vi "WriteScript.vi"(0 "X1":dbl[](array[numeric]), 1 "Y1":dbl[](array[numeric]), 2 "X2":dbl[](array[numeric]), 3 "Y2":dbl[](array[numeric]), 4 "Pause":i32, 5 "C0":i32, 6 "C1":i32, 7 "error in":errorcluster, 9 "Seq":string) -> (20 "concatenated string":string, 27 "error out":errorcluster)   [LabVIEW 2017]
panel:
  out "B2":dbl
  out "G2":dbl
  out "R2":dbl
  out "Resolved Color 2":u32 format="%.0x"
  out "B1":dbl
  out "G1":dbl
  out "R1":dbl
  out "Resolved Color 1":u32 format="%.0x"
  # "M. Zemp & I. Scholl GM BA 2"
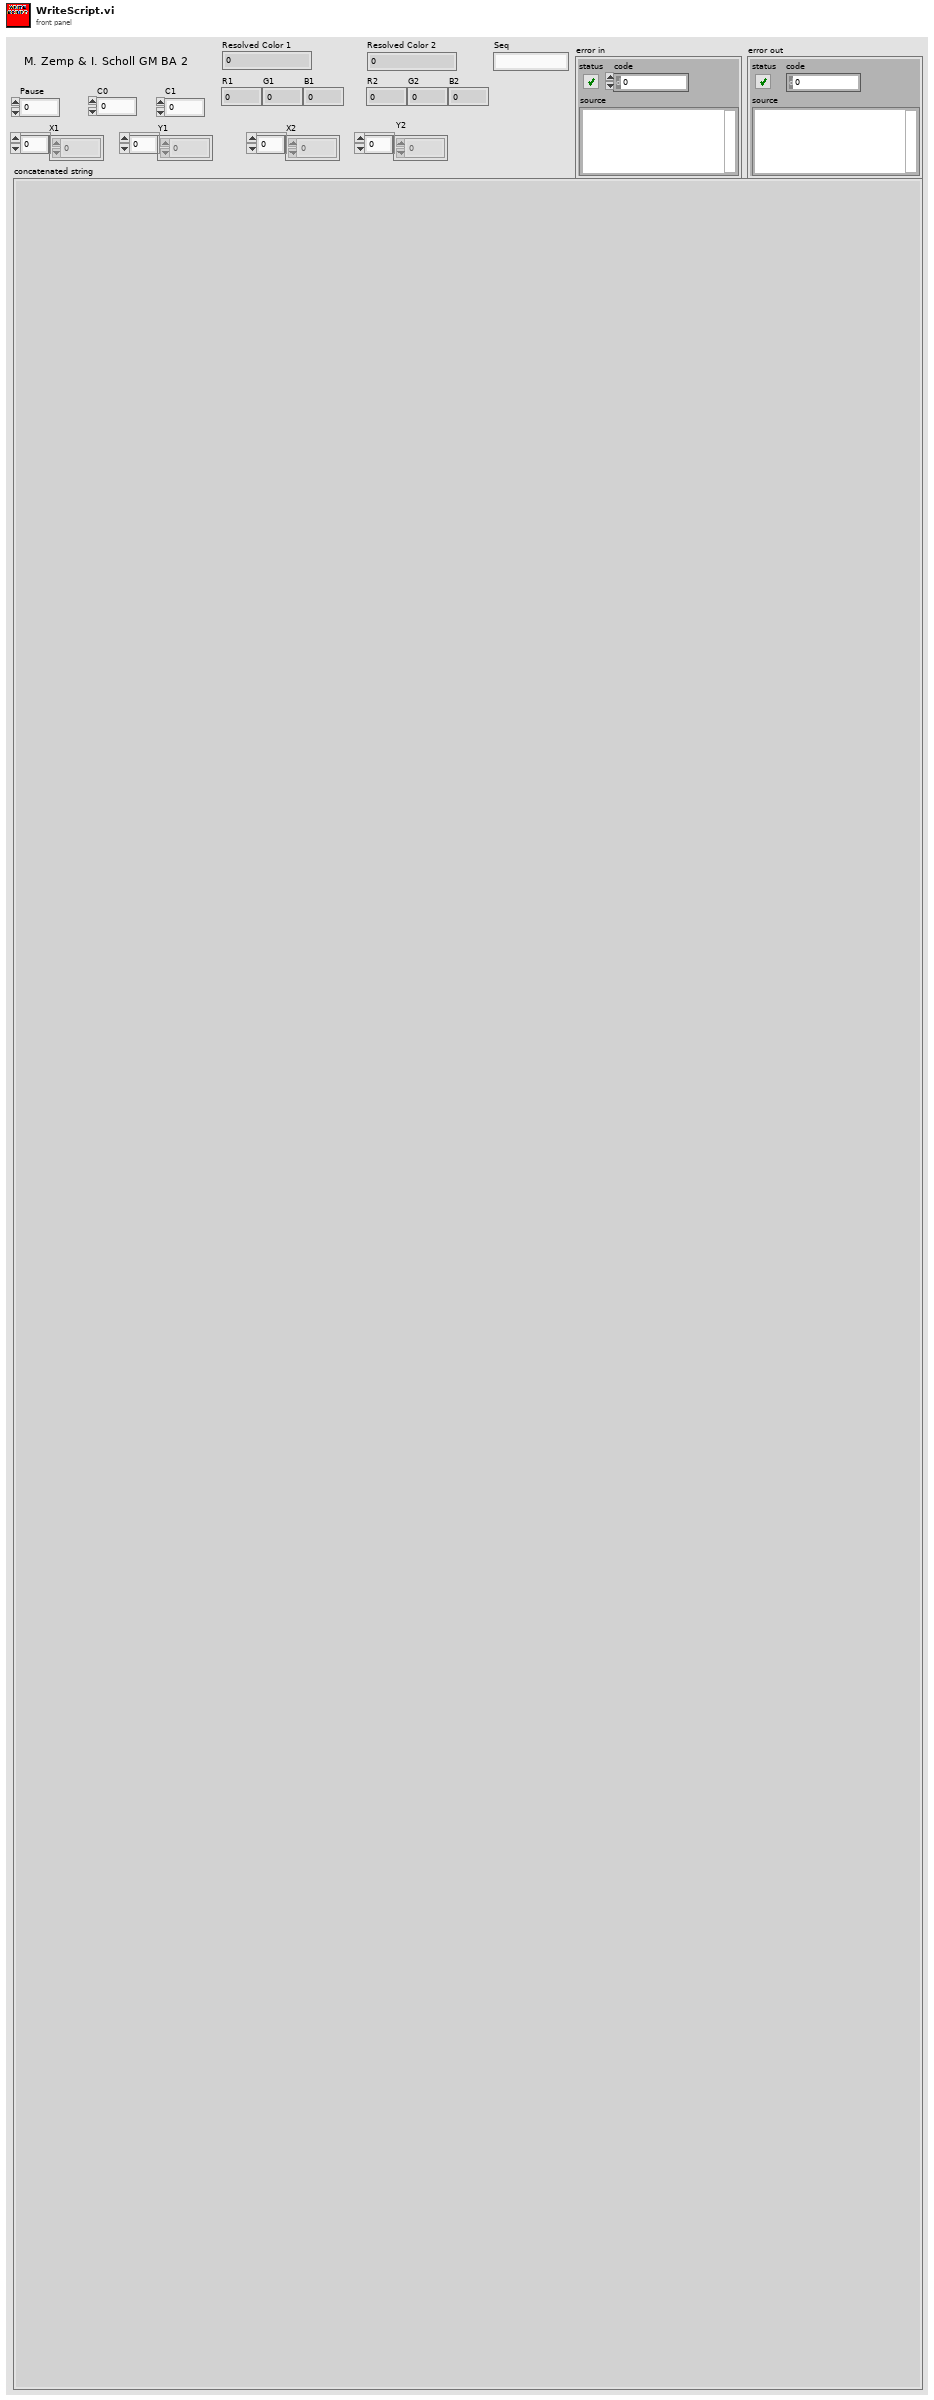
[diagram p1: front panel]
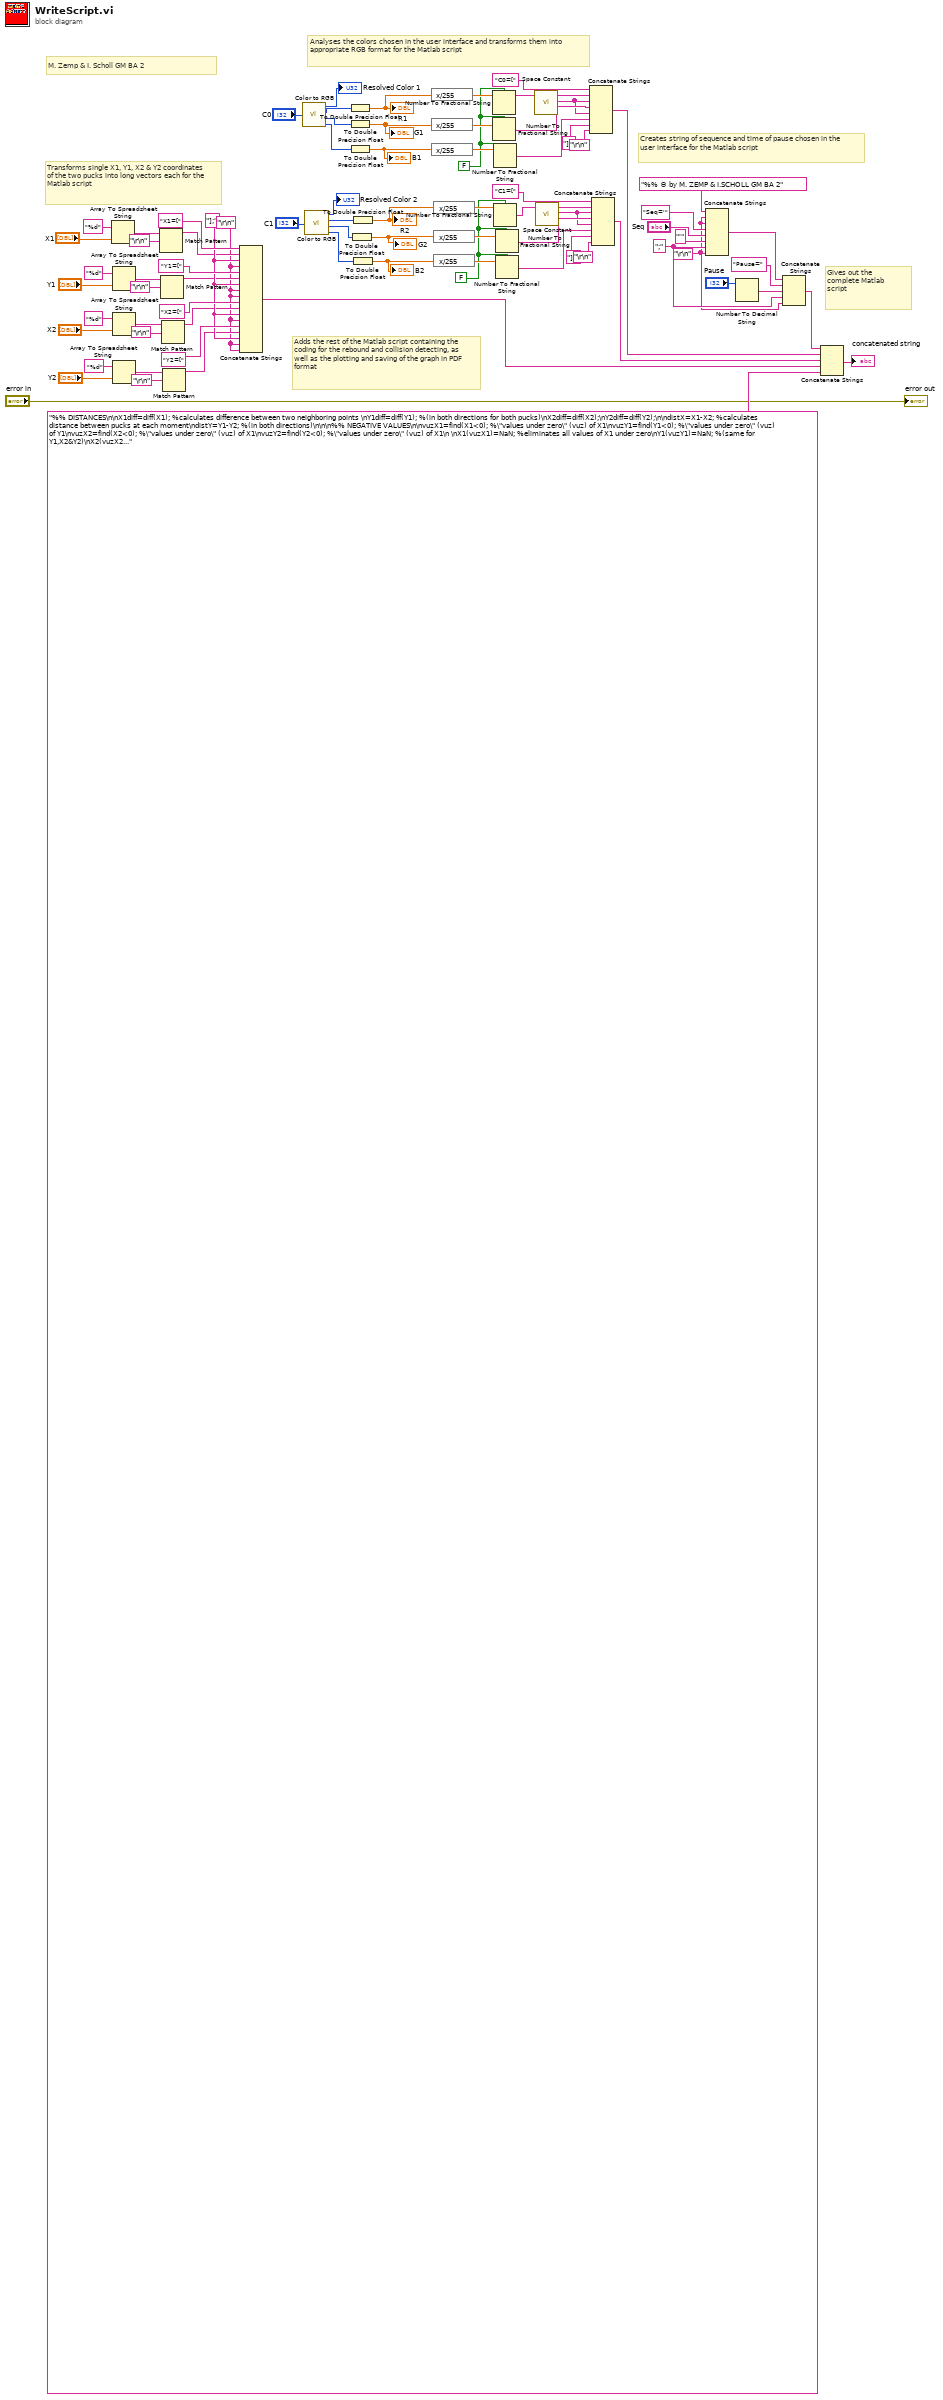
[diagram p0: block diagram]
diagram:
  w5 = FALSE
  w6 = FALSE ("use system decimal point (T)")
  w1 = "\r\n"
  w9 = ";"
  w4 = "\r\n"
  w73 = "];"
  # "M. Zemp & I. Scholl GM BA 2"
  # "Adds the rest of the Matlab script containing the coding for the rebound and collision detecting, as well as the plotting and saving of the graph in PDF format"
  # "Gives out the complete Matlab script"
  # "Creates string of sequence and time of pause chosen in the user interface for the Matlab script"
  # "Analyses the colors chosen in the user interface and transforms them into appropriate RGB format for the Matlab script"
  # "Transforms single X1, Y1, X2 & Y2 coordinates of the two pucks into long vectors each for the Matlab script"
  n1 = Array To Spreadsheet String(array="X1", 3:"%d" ("format string")) -> (spreadsheet string=w72:string)  [unwired: 1 in]
  n2 = Array To Spreadsheet String(array="Y1", 3:"%d" ("format string")) -> (spreadsheet string=w64:string)  [unwired: 1 in]
  n3 = Array To Spreadsheet String(array="X2", 3:"%d" ("format string")) -> (spreadsheet string=w61:string)  [unwired: 1 in]
  n4 = Array To Spreadsheet String(array="Y2", 3:"%d" ("format string")) -> (spreadsheet string=w58:string)  [unwired: 1 in]
  n5 = Match Pattern(string=w72, regular expression="\r\n") -> (before substring=w66:string)  [unwired: 1 in, 3 out]
  n6 = Match Pattern(string=w64, regular expression="\r\n") -> (before substring=w63:string)  [unwired: 1 in, 3 out]
  n7 = Match Pattern(string=w61, regular expression="\r\n") -> (before substring=w60:string)  [unwired: 1 in, 3 out]
  n8 = Match Pattern(string=w58, regular expression="\r\n") -> (before substring=w57:string)  [unwired: 1 in, 3 out]
  n9 = Concatenate Strings("X1=[", w66, w73, w4, "Y1=[", w63, w73, w4, w4, "X2=[", w60, w73, w4, "Y2=[", w57, w73, w4, w4) -> (w56:string)
  n10 = call <vilib>:"Color to RGB.vi"("Color"="C0") -> ("Resolved Color"=→"Resolved Color 1":u32, "R"=w44:u8, "G"=w43:u8, "B"=w42:u8)
  n11 = call <vilib>:"Color to RGB.vi"("Color"="C1") -> ("Resolved Color"=→"Resolved Color 2":u32, "R"=w25:u8, "G"=w24:u8, "B"=w23:u8)
  n12 = To Double Precision Float(number=w44) -> (double precision float=w39:dbl)
  "R1" <- w39
  n13 = To Double Precision Float(number=w43) -> (double precision float=w40:dbl)
  "G1" <- w40
  n14 = To Double Precision Float(number=w42) -> (double precision float=w41:dbl)
  "B1" <- w41
  n15 = To Double Precision Float(number=w24) -> (double precision float=w21:dbl)
  "G2" <- w21
  n16 = To Double Precision Float(number=w25) -> (double precision float=w20:dbl)
  "R2" <- w20
  n17 = To Double Precision Float(number=w23) -> (double precision float=w22:dbl)
  "B2" <- w22
  n18 = expression code="x/255"(w39) -> (w45:dbl)
  n19 = expression code="x/255"(w40) -> (w48:dbl)
  n20 = expression code="x/255"(w41) -> (w47:dbl)
  n21 = expression code="x/255"(w20) -> (w30:dbl)
  n22 = expression code="x/255"(w21) -> (w29:dbl)
  n23 = expression code="x/255"(w22) -> (w28:dbl)
  n24 = Number To Fractional String(use system decimal point (T)=w6, number=w45) -> (F-format string=w7:string)  [unwired: 2 in]
  n25 = Number To Fractional String(use system decimal point (T)=w6, number=w48) -> (F-format string=w34:string)  [unwired: 2 in]
  n26 = Number To Fractional String(use system decimal point (T)=w6, number=w47) -> (F-format string=w33:string)  [unwired: 2 in]
  n27 = Number To Fractional String(use system decimal point (T)=w5, number=w30) -> (F-format string=w26:string)  [unwired: 2 in]
  n28 = Number To Fractional String(use system decimal point (T)=w5, number=w29) -> (F-format string=w17:string)  [unwired: 2 in]
  n29 = Number To Fractional String(use system decimal point (T)=w5, number=w28) -> (F-format string=w16:string)  [unwired: 2 in]
  n30 = call <vilib>:"Space Constant.vi"() -> ("String"=w32:string)
  n31 = call <vilib>:"Space Constant.vi"() -> ("String"=w15:string)
  n32 = Concatenate Strings("C0=[", w7, w32, w34, w32, w33, "];", "\r\n") -> (w35:string)
  n33 = Concatenate Strings("C1=[", w26, w15, w17, w15, w16, "];", "\r\n") -> (w13:string)
  n34 = Concatenate Strings("%% © by M. ZEMP & I.SCHOLL GM BA 2", w1, w1, "Seq='", "Seq", "'", w9, w1) -> (w10:string)
  n35 = Number To Decimal String(number="Pause") -> (decimal integer string=w51:string)  [unwired: 1 in]
  n36 = Concatenate Strings(w10, "Pause=", w51, w9, w1) -> (w36:string)
  n37 = Concatenate Strings(w36, w35, w13, w56, "%% DISTANCES\n\nX1diff=diff(X1); %calculates difference between two neighboring points \nY1diff=diff(Y1); %(in both directions for both pucks)\nX2diff=diff(X2);\nY2diff=diff(Y2);\n\ndistX=X1-X2; %calculates distance between pucks at each moment\ndistY=Y1-Y2; %(in both directions)\n\n\n%% NEGATIVE VALUES\n\nvuzX1=find(X1<0); %\"values under zero\" (vuz) of X1\nvuzY1=find(Y1<0); %\"values under zero\" (vuz) of Y1\nvuzX2=find(X2<0); %\"values under zero\" (vuz) of X1\nvuzY2=find(Y2<0); %\"values under zero\" (vuz) of X1\n \nX1(vuzX1)=NaN; %eliminates all values of X1 under zero\nY1(vuzY1)=NaN; %(same for Y1,X2&Y2)\nX2(vuzX2)=NaN;\nY2(vuzY2)=NaN;\n\n\n%% MIN/MAX VALUES\n\nXmin=min([X1 X2]); %calculates minimal and maximal value in each direction\nXmax=max([X1 X2]);\nYmin=min([Y1 Y2]);\nYmax=max([Y1 Y2]);\n\n\n%% BORDER REBOUNDS\n\nrB=15;\n\nrebX1max=find(X1+rB>=Xmax); % calculates rebounds with right border of puck 1\nCtrlX1max=[0 rebX1max];\nCtrlX1max=([rebX1max 0]-CtrlX1max==1);\nCtrlX1max(end)=[];\nrebX1max=rebX1max-rebX1max.*CtrlX1max;\nrebX1max(find(rebX1max==0))=[];\n\nrebX1min=find(X1-rB<=Xmin); % calculates rebounds with left border of puck 1\nCtrlX1min=[0 rebX1min];\nCtrlX1min=([rebX1min 0]-CtrlX1min==1);\nCtrlX1min(end)=[];\nrebX1min=rebX1min-rebX1min.*CtrlX1min;\nrebX1min(find(rebX1min==0))=[];\n\nrebY1max=find(Y1+rB>=Ymax); % calculates rebounds with top border of puck 1\nCtrlY1max=[0 rebY1max];\nCtrlY1max=([rebY1max 0]-CtrlY1max==1);\nCtrlY1max(end)=[];\nrebY1max=rebY1max-rebY1max.*CtrlY1max;\nrebY1max(find(rebY1max==0))=[];\n\nrebY1min=find(Y1-rB<=Ymin); % calculates rebounds with bottom border of puck 1\nCtrlY1min=[0 rebY1min];\nCtrlY1min=([rebY1min 0]-CtrlY1min==1);\nCtrlY1min(end)=[];\nrebY1min=rebY1min-rebY1min.*CtrlY1min;\nrebY1min(find(rebY1min==0))=[];\n\n\nrebX2max=find(X2+rB>=Xmax); % calculates rebounds with right border of puck 2\nCtrlX2max=[0 rebX2max];\nCtrlX2max=([rebX2max 0]-CtrlX2max==1);\nCtrlX2max(end)=[];\nrebX2max=rebX2max-rebX2max.*CtrlX2max;\nrebX2max(find(rebX2max==0))=[];\n\nrebX2min=find(X2-rB<=Xmin); % calculates rebounds with left border of puck 2\nCtrlX2min=[0 rebX2min];\nCtrlX2min=([rebX2min 0]-CtrlX2min==1);\nCtrlX2min(end)=[];\nrebX2min=rebX2min-rebX2min.*CtrlX2min;\nrebX2min(find(rebX2min==0))=[];\n\nrebY2max=find(Y2+rB>=Ymax); % calculates rebounds with top border of puck 2\nCtrlY2max=[0 rebY2max];\nCtrlY2max=([rebY2max 0]-CtrlY2max==1);\nCtrlY2max(end)=[];\nrebY2max=rebY2max-rebY2max.*CtrlY2max;\nrebY2max(find(rebY2max==0))=[];\n\nrebY2min=find(Y2-rB<=Ymin); % calculates rebounds with bottom border of puck 2\nCtrlY2min=[0 rebY2min];\nCtrlY2min=([rebY2min 0]-CtrlY2min==1);\nCtrlY2min(end)=[];\nrebY2min=rebY2min-rebY2min.*CtrlY2min;\nrebY2min(find(rebY2min==0))=[];\n\n\n%% PUCK COLLISIONS\n\nDmin=50; %settings for collision\nalphamin=1;\npos=1:length(X1);\n\nP1ang1=atan2(Y1diff,X1diff); %calculates angle of movement of puck 1\nP1ang2=[0 P1ang1];\nP1ang2(end)=[];\nP1ang3=abs(P1ang2-P1ang1);\n\n \npos(find(P1ang3<alphamin))=0; %finds all puck collisions\npos(find(sqrt(distX.^2.+distY.^2)>Dmin))=0;\npos(intersect(pos,find(Y1+rB>=Ymax)))=0; %eliminates rebound positions\npos(intersect(pos,find(Y2+rB>=Ymax)))=0;\npos(intersect(pos,find(X1+rB>=Xmax)))=0;\npos(intersect(pos,find(X2+rB>=Xmax)))=0;\npos(intersect(pos,find(Y1-rB<=Ymin)))=0;\npos(intersect(pos,find(Y2-rB<=Ymin)))=0;\npos(intersect(pos,find(X1-rB<=Xmin)))=0;\npos(intersect(pos,find(X2-rB<=Xmin)))=0;\n\npos(find(pos==0))=[];\n\n\n%% PLOTTING\n\nfigure(); %starts plotting of graphs\nhold on; \naxis([-10 615 -50 440]); %sets axes\ndaspect([1.2 1 1]); %sets ratio between data steps on axes\nrectangle('Position',[Xmin Ymin Xmax-Xmin Ymax-Ymin]); %creates borders of AirHockey-table\nP1=plot(X1,Y1,'-','LineWidth',1); %plots the graph for Puck 1\nP2=plot(X2,Y2,'-','LineWidth',1); %plots the graph for Puck 2\nset(P1,'Marker','.','MarkerSize',17,'Color',C0); %sets properties of Puck 1's graph\nset(P2,'Marker','.','MarkerSize',17,'Color',C1); %sets properties of Puck 2's graph\n\ntitle('Air Hockey','FontSize',20); %writes title\n\nrebP1=scatter(X1(rebX1max),Y1(rebX1max),100,'MarkerEdgeColor',C0); % plots all collisions with borders\nscatter(X1(rebX1min),Y1(rebX1min),100,'MarkerEdgeColor',C0);\nscatter(X1(rebY1max),Y1(rebY1max),100,'MarkerEdgeColor',C0); \nscatter(X1(rebY1min),Y1(rebY1min),100,'MarkerEdgeColor',C0);\nrebP2=scatter(X2(rebX2max),Y2(rebX2max),100,'MarkerEdgeColor',C1); \nscatter(X2(rebX2min),Y2(rebX2min),100,'MarkerEdgeColor',C1);\nscatter(X2(rebY2max),Y2(rebY2max),100,'MarkerEdgeColor',C1); \nscatter(X2(rebY2min),Y2(rebY2min),100,'MarkerEdgeColor',C1);\n\ncoll=scatter(X1(pos),Y1(pos),400,'r','MarkerFaceColor','r','MarkerFaceAlpha',0.2); %,'MarkerSize',11,'MarkerEdgeColor','r','MarkerFaceColor','r','LineWidth',2); % plots puck collisions\nscatter(X2(pos),Y2(pos),400,'r','MarkerFaceColor','r','MarkerFaceAlpha',0.2);\n\n\nd = datetime('now'); %writes current date&time\ntext(130,330,string(d));    \n\nBTP1=length(rebX1max)+length(rebX1min)+length(rebY1max)+length(rebY1min); %writes number of rebounds of puck 1\nBTP1Str=strcat(string(BTP1),' band(s) touched by puck 1');\ntext(40,15,BTP1Str);\n\nBTP2=length(rebX2max)+length(rebX2min)+length(rebY2max)+length(rebY2min); %writes number of rebounds of puck 2\nBTP2Str=strcat(string(BTP2),' band(s) touched by puck 2');\ntext(40,-5,BTP2Str);\n\nNrCol=length(pos); %writes number of puck collisions\nColStr=strcat(string(NrCol),' puck collision(s)');\ntext(40,-25,ColStr);\n\ntext(40,330,Seq); %writes sequence name\n\ntext(400,-25,'© by M.Zemp, I. Scholl GM BA2','FontSize',6) % writes authors names\n\nlegend([P1 P2 rebP1 rebP2 coll],'puck 1','puck 2','rebound puck 1','rebound puck 2','puck collision'); %creates graphic's legend\nlegend('boxoff'); %takes away frame from legend box\n\nhold off;\n\n\n%% DISPLAYING AND SAVING\n\npause(Pause);\n\nsaveas(gcf,'AH_score.pdf','pdf'); %saves plot as PDF document") -> (→"concatenated string":string)
  "error out" <- "error in"
